vi "Q_selecter.vi"(8 "String 2":string="C:\\Users\\dalek669528\\Desktop\\CNC_proj\\workspace\\data\\X_Q_0426.csv", 9 "Numeric 5":i32, 10 "String":string="C:\\Users\\dalek669528\\Desktop\\CNC_proj\\workspace\\data\\X_Q_0426.csv", 11 "Numeric 4":i32) -> (0 "Boolean 3":bool, 1 "Array 2":dbl[](array[numeric]), 2 "Boolean 2":bool, 3 "Array":dbl[](array[numeric]))   [LabVIEW 2019]
uses:
  <vilib>/Analysis/Matrix/Datatypes/RealMatrix.ctl
  <vilib>/Utility/file.llb/Write Delimited Spreadsheet (DBL).vi
  <vilib>/Utility/file.llb/Read Delimited Spreadsheet (DBL).vi
  <vilib>/Analysis/Matrix/NI_Matrix.lvlib
panel:
  out "Numeric 7":dbl
  out "Numeric 6":dbl
  out "Real Matrix\n 2":T1
  out "Numeric 3":dbl
  in  "Boolean":bool=TRUE
  out "Numeric 2":dbl
  out "Numeric":dbl
  out "Real Matrix":T1
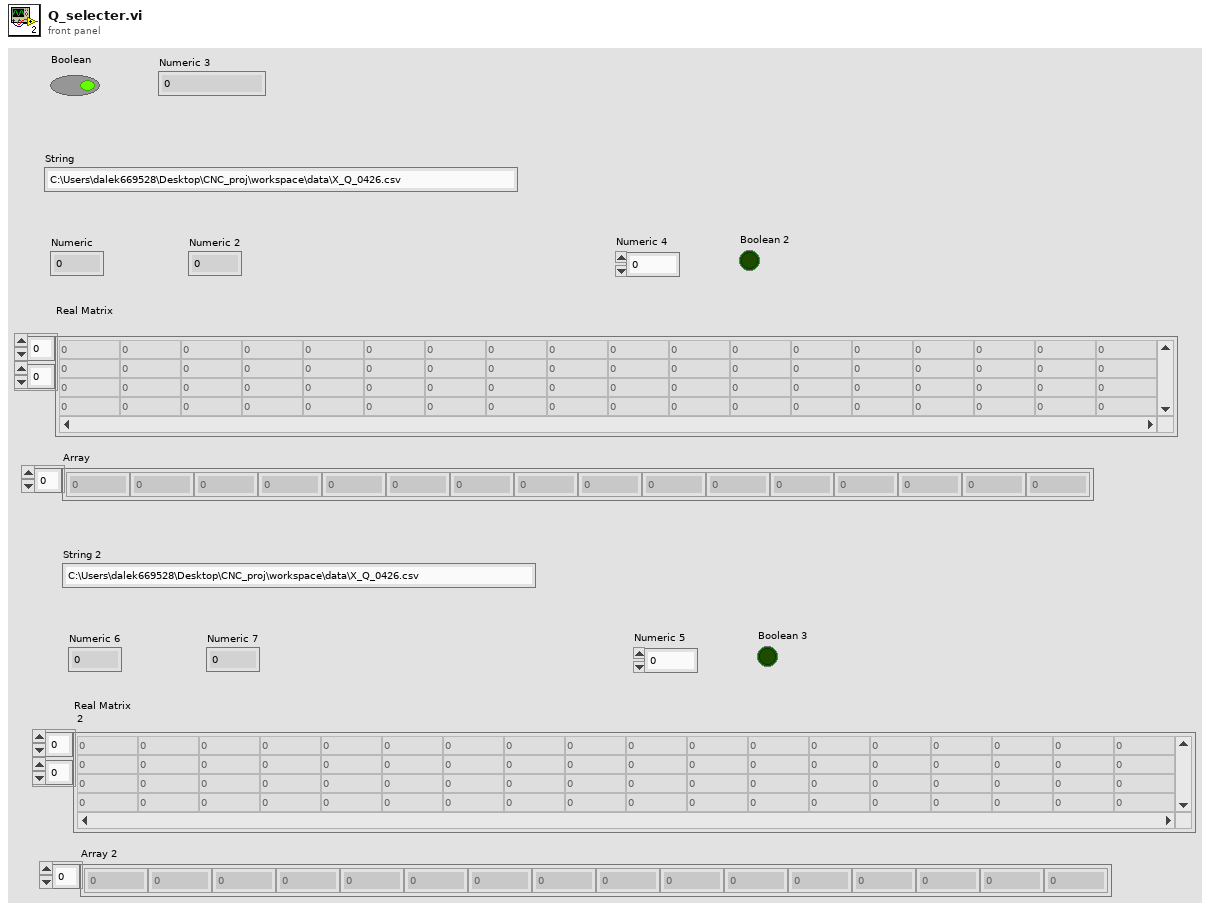
[diagram p1: front panel]
types:
  T1 = typedef "NI_Matrix.lvlib/RealMatrix.ctl" = dbl[][]
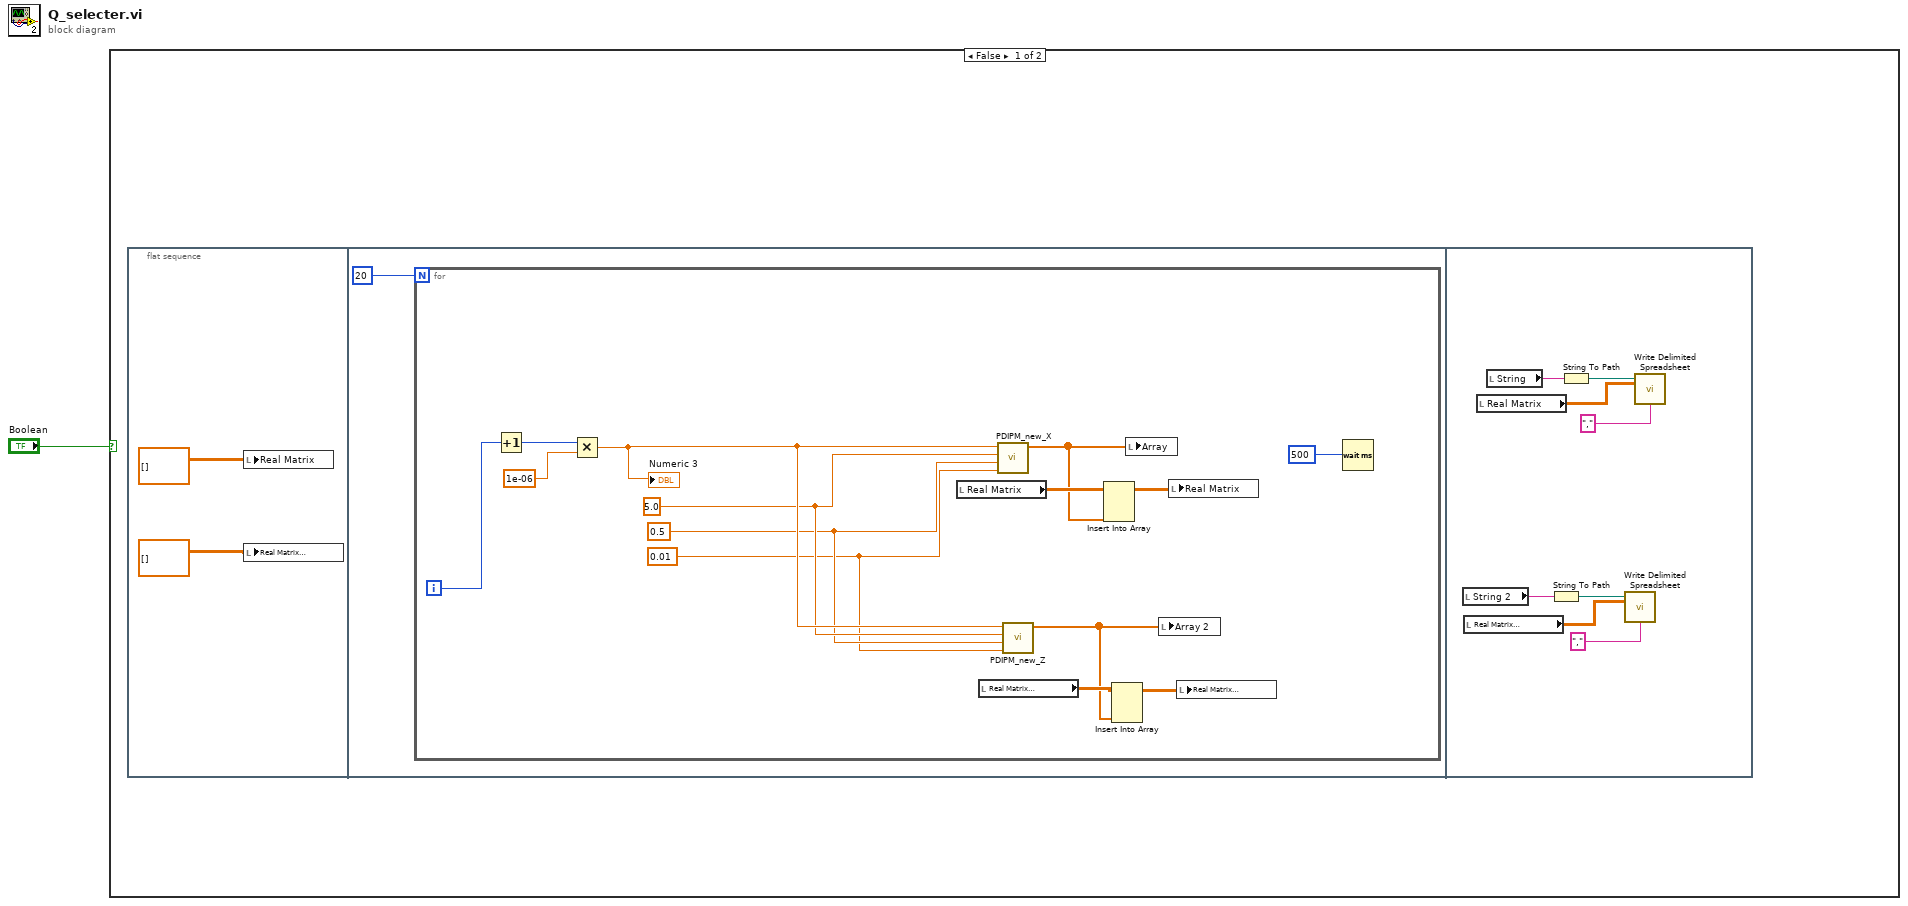
[diagram p0: block diagram]
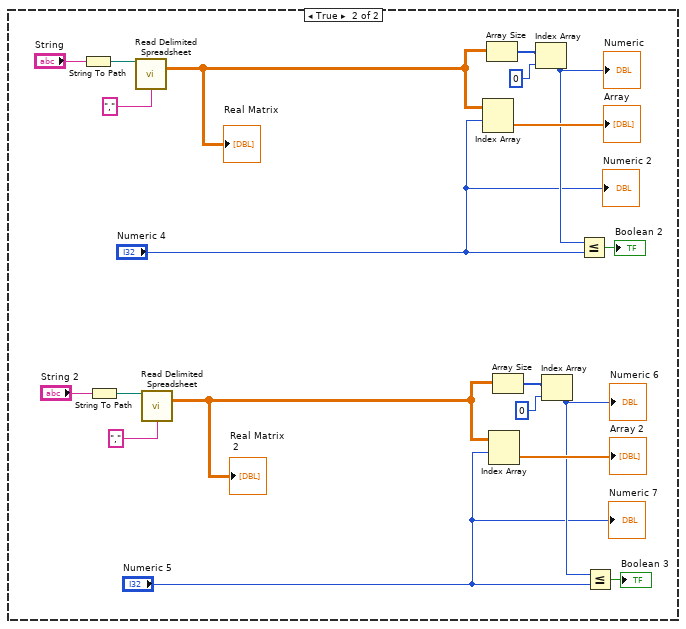
[diagram p2: hidden frame]
diagram:
  n1 = case shown="False" "Boolean" {
    frame False {
      n2 = flat-sequence {
        frame #0 {
          n3 = local write "Real Matrix"(dbl[][] []) -> ()
          n4 = local write "Real Matrix\n 2"(dbl[][] []) -> ()
        }
        frame #1 {
          n5 = for {
            N: 20 -> [_]
            i -> [w18]
            w8 = 0.01
            w9 = 0.5
            w10 = 5.0
            n6 = Increment(x=w18) -> (x+1=w16:i32)
            n7 = Multiply(x=w16, y=1e-06) -> (x*y=w11:dbl)
            "Numeric 3" <- w11
            n8 = local read "Real Matrix"() -> (w15:T1)
            n9 = local read "Real Matrix\n 2"() -> (w7:T1)
            n10 = call "PDIPM_new_X.vi"("alpha"=w8, "beta"=w9, "m_mu"=w10, "convergence\ncriterion"=w11) -> ("Q_num"=w14:dbl[])  [unwired: 6 in, 1 out]
            n11 = call "PDIPM_new_Z.vi"("alpha"=w8, "beta"=w9, "m_mu"=w10, "convergence\ncriterion"=w11) -> ("Q_num"=w5:dbl[])  [unwired: 6 in, 1 out]
            n12 = Insert Into Array(array=w15, new element=w14) -> (w13:T1)  [unwired: 2 in]
            n13 = Insert Into Array(array=w7, new element=w5) -> (w6:T1)  [unwired: 2 in]
            n14 = local write "Array"(w14) -> ()
            n15 = local write "Array 2"(w5) -> ()
            n16 = local write "Real Matrix"(w13) -> ()
            n17 = local write "Real Matrix\n 2"(w6) -> ()
            n18 = Wait (ms)(milliseconds to wait=500) -> ()  [unwired: 1 out]
          }
        }
        frame #2 {
          n19 = local read "String 2"() -> (w20:string)
          n20 = local read "Real Matrix\n 2"() -> (w19:T1)
          n21 = local read "Real Matrix"() -> (w23:T1)
          n22 = local read "String"() -> (w26:string)
          n23 = String To Path(string=w20) -> (path=w22:path)
          n24 = String To Path(string=w26) -> (path=w25:path)
          n25 = call-poly <vilib>:"Write Delimited Spreadsheet.vi"("file path (dialog if empty)"=w22, "2D data"=w19, "delimiter (\\t)"=",") -> ()  [unwired: 11 in, 2 out]
          n26 = call-poly <vilib>:"Write Delimited Spreadsheet.vi"("file path (dialog if empty)"=w25, "2D data"=w23, "delimiter (\\t)"=",") -> ()  [unwired: 11 in, 2 out]
        }
      }
    }
    frame True {
      n27 = String To Path(string="String") -> (path=w44:path)
      n28 = String To Path(string="String 2") -> (path=w34:path)
      n29 = call-poly <vilib>:"Read Delimited Spreadsheet.vi"("file path (dialog if empty)"=w44, "delimiter (\\t)"=",") -> ("all rows"=w46:dbl[][])  [unwired: 8 in, 5 out]
      "Real Matrix" <- w46
      n30 = call-poly <vilib>:"Read Delimited Spreadsheet.vi"("file path (dialog if empty)"=w34, "delimiter (\\t)"=",") -> ("all rows"=w36:dbl[][])  [unwired: 8 in, 5 out]
      "Real Matrix\n 2" <- w36
      n31 = Index Array(array=w46, index (row)="Numeric 4") -> (element=→"Array":dbl[])  [unwired: 1 in]
      n32 = Array Size(array=w46) -> (size(s)=w41:i32[])
      n33 = Index Array(array=w36, index (row)="Numeric 5") -> (element=→"Array 2":dbl[])  [unwired: 1 in]
      n34 = Array Size(array=w36) -> (size(s)=w31:i32[])
      n35 = Index Array(array=w41, index=0) -> (element=w38:i32)
      "Numeric" <- w38
      n36 = Index Array(array=w31, index=0) -> (element=w28:i32)
      "Numeric 6" <- w28
      n37 = Less Or Equal?(x=w38, y="Numeric 4") -> (x <= y?=→"Boolean 2":bool)
      n38 = Less Or Equal?(x=w28, y="Numeric 5") -> (x <= y?=→"Boolean 3":bool)
      "Numeric 2" <- "Numeric 4"
      "Numeric 7" <- "Numeric 5"
    }
  }
